vi "setTensao.vi"(7 "Numeric":i32, 8 "error in (no error)":errorcluster, 9 "Pontos":dbl, 10 "Tensão máxima":dbl, 11 "delay(s)":dbl) -> (0 "error out":errorcluster, 2 "output voltage":dbl, 3 "output voltage 2":dbl)   [LabVIEW 2012]
uses:
  <instrlib>/Agilent 6XXX Series/Agilent 6XXX Series.lvlib
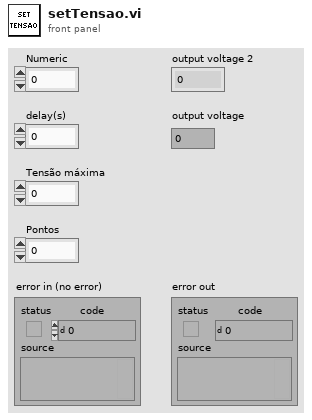
[diagram p1: front panel]
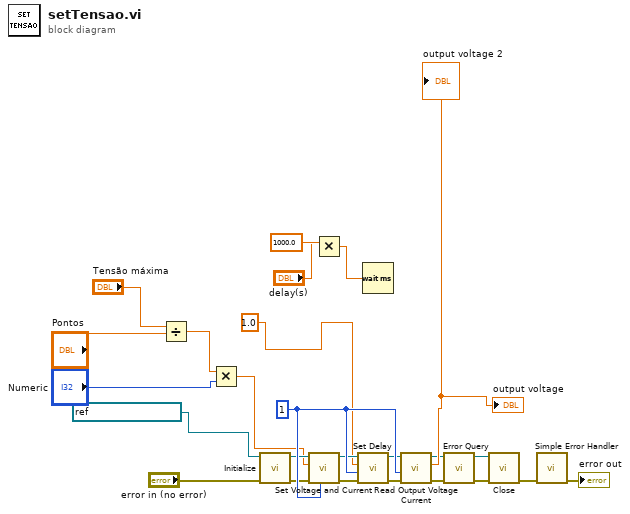
[diagram p0: block diagram]
diagram:
  w18 = u8 1 ("channel (1)")
  n1 = Divide(x="Tensão máxima", y="Pontos") -> (x/y=w17:dbl)
  n2 = Multiply(x=w17, y="Numeric") -> (x*y=w5:dbl)
  n3 = call <instrlib>:"Initialize.vi"("error in (no error)"="error in (no error)", "VISA resource name"=refnum<visa-resource-name> "GPIB0::5::INSTR") -> ("error out"=w11:errorcluster, "VISA resource name out"=w12:refnum<visa-resource-name>)  [unwired: 8 in]
  n4 = call <instrlib>:"Set Voltage and Current.vi"("channel (1)"=w18, "error in (no error)"=w11, "voltage (0 V)"=w5, "VISA resource name"=w12) -> ("error out"=w7:errorcluster, "VISA resource name out"=w6:refnum<visa-resource-name>)  [unwired: 6 in]
  n5 = Multiply(x="delay(s)", y=1000.0) -> (x*y=w22:dbl)
  n6 = call <instrlib>:"Set Delay.vi"("error in (no error)"=w7, "channel (1)"=w18, "delay (0 s)"=1.0, "VISA resource name"=w6) -> ("error out"=w3:errorcluster, "VISA resource name out"=w4:refnum<visa-resource-name>)  [unwired: 6 in]
  n7 = Wait (ms)(milliseconds to wait=w22) -> ()  [unwired: 1 out]
  n8 = call <instrlib>:"Read Output Voltage Current.vi"("error in (no error)"=w3, "channel (1)"=w18, "VISA resource name"=w4) -> ("error out"=w9:errorcluster, "output voltage"=→"output voltage" →"output voltage 2":dbl, "VISA resource name out"=w8:refnum<visa-resource-name>)  [unwired: 5 in, 1 out]
  n9 = call <instrlib>:"Error Query.vi"("error in (no error)"=w9, "VISA resource name"=w8) -> ("error out"=w14:errorcluster, "VISA resource name out"=w13:refnum<visa-resource-name>)  [unwired: 6 in, 2 out]
  n10 = call <instrlib>:"Close.vi"("error in (no error)"=w14, "VISA resource name"=w13) -> ("error out"=w15:errorcluster)  [unwired: 9 in]
  n11 = call <vilib>:"Simple Error Handler.vi"("error in (no error)"=w15) -> ("error out"=→"error out":errorcluster)  [unwired: 4 in, 4 out]
